vi "read.vi"(8 "error in":errorcluster, 9 "timeout in ms (-1)":i32=-1, 11 "stream publisher in":refnum<class "data bus stream subscriber.lvclass">) -> (0 "error out":errorcluster, 1 "timed out?":bool, 2 "element":T1, 3 "stream publisher out":refnum<class "data bus stream subscriber.lvclass">)   [LabVIEW 2013, in "data bus stream subscriber.lvclass"]
uses:
  data bus stream subscriber.lvclass
  data stream definition.ctl
  data stream message type.ctl
  data bus stream subscriber.lvclass/data bus stream subscriber.ctl
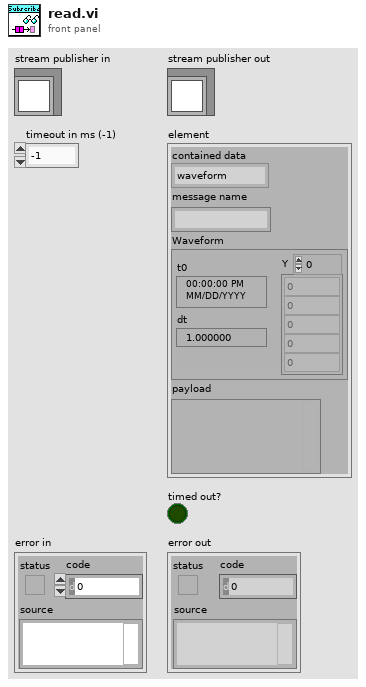
[diagram p1: front panel]
types:
  T1 = typedef "data stream definition.ctl" = cluster{"contained data":T2, "message name":string, "Waveform":waveform(dbl), "payload":variant}
  T2 = typedef "data stream message type.ctl" = enum16{"waveform", "message"}
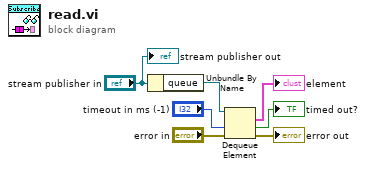
[diagram p0: block diagram]
diagram:
  n1 = Unbundle By Name("stream publisher in") -> ("queue"=w4:refnum<queue>)
  n2 = Dequeue Element(queue=w4, timeout in ms (-1)="timeout in ms (-1)", error in (no error)="error in") -> (element=→"element":T1, timed out?=→"timed out?":bool, error out=→"error out":errorcluster)  [unwired: 1 out]
  "stream publisher out" <- "stream publisher in"
